vi "Write ErrorColorBG.vi"(8 "error in":errorcluster, 10 "ErrorColorBG":u32(colorbox), 11 "EmailField in":refnum<class "EmailField.lvclass">) -> (0 "error out":errorcluster, 3 "EmailField out":refnum<class "EmailField.lvclass">)   [LabVIEW 2020, in "EmailField.lvclass"]
uses:
  EmailField.lvclass
  EmailField.lvclass/EmailField.ctl
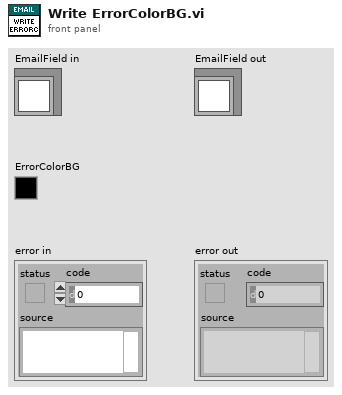
[diagram p1: front panel]
types:
  T1 = typedef "EmailField.lvclass/State Data.ctl" = cluster{"CorrectColorBG":u32, "CorrectColorText":u32, "ErrorColorBG":u32, "ErrorColorText":u32}
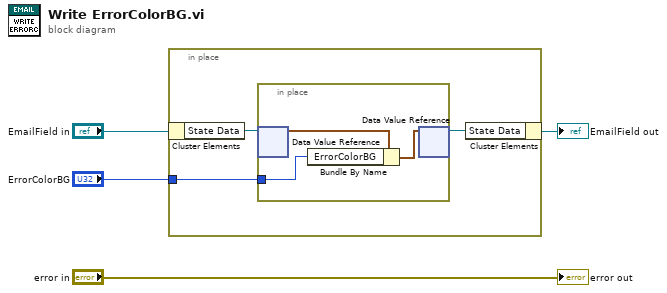
[diagram p0: block diagram]
diagram:
  n1 = in-place {
    in-place-border: "ErrorColorBG" -> [w5]
    n2 = in-place-cluster #1("EmailField in") -> ("State Data"=w7:refnum<data-value>)
    n3 = in-place {
      in-place-border: w5 -> [w8]
      n4 = in-place-dvr #2(w7) -> (w10:T1)  [unwired: 1 out]
      n5 = Bundle By Name(cluster=w10, "ErrorColorBG"=w8) -> (w9:T1)
      n6 = in-place-dvr #2(w9) -> (w6:refnum<data-value>)  [unwired: 1 out]
    }
    n7 = in-place-cluster #1("State Data"=w6) -> (→"EmailField out":refnum<class "EmailField.lvclass">)
  }
  "error out" <- "error in"
